vi "Read_input.vi"(11 "L       E \nIndicator":T1 caption="L      E") -> (3 "Input":u16)   [LabVIEW 2023]
uses:
  controls/Boolean L E indictaor.ctl
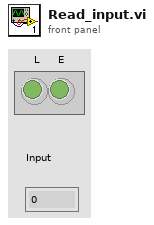
[diagram p1: front panel]
types:
  T1 = typedef "Boolean L E indictaor.ctl" = bool[]
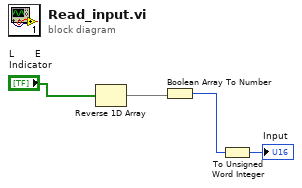
[diagram p0: block diagram]
diagram:
  n1 = Reverse 1D Array(array="L       E \nIndicator") -> (reversed array=w2:T1)
  n2 = Boolean Array To Number(Boolean array=w2) -> (number=w3:u32)
  n3 = To Unsigned Word Integer(number=w3) -> (unsigned 16bit integer=→"Input":u16)
